vi "new encoder trial.vi"() -> ()   [LabVIEW 2018]
uses:
  <vilib>/Platform/TimedLoop/XDataNode/timing_clust.ctl
  <vilib>/Platform/TimedLoop/XDataNode/nitl_modes.ctl
  <vilib>/Platform/TimedLoop/XDataNode/wakeup.ctl
  <vilib>/rvi/eio/common/nirviEmuTemplateMethod_errors.vi
  <vilib>/rvi/Emulation/niFpgaGetClockAttributes.vi
  <vilib>/rvi/Emulation/niFpgaSctlEmulationGetInTimedLoop.vi
  <vilib>/rvi/Emulation/niFpgaEmulationReportErrorSimple.vi
  <vilib>/rvi/Emulation/niFpgaCriticalErrorInLSC.vi
  <vilib>/eio/EIOMethodNode/EIOMethodNode.xnode
  <vilib>/eio/EIONode/EIONode.xnode
  <vilib>/platform/TimedLoop/XDataNode/XDataNode.xnode
  <vilib>/Platform/TimedLoop/XDataNode/XDNodeRunTimeDep.lvlib
panel:
  out "Mod7/DIO1":bool
  out "Mod7/DIO0":bool
  out "appended array":sgl[](array[numeric])
  out "edge detected":bool
  in  "falling edge (F)":bool caption="Torque encoder direction"
  in  "switch encoders":bool
  in  "filterTorque":bool
  in  "encoders offset":sgl caption="encoder offset (radians)"
  in  "Digital Out":bool[](array[boolean])=[FALSE, FALSE, FALSE, FALSE, FALSE, FALSE, FALSE, FALSE]
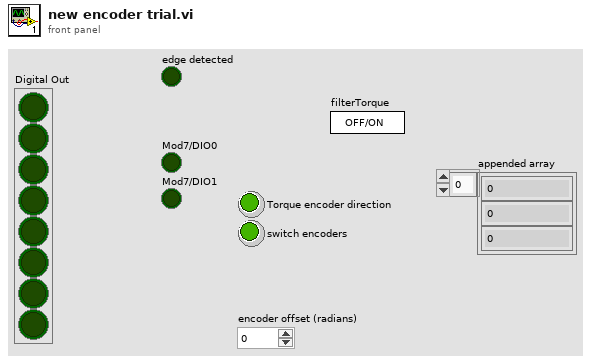
[diagram p1: front panel]
types:
  T1 = typedef "XDNodeRunTimeDep.lvlib/timing_clust.ctl" = cluster{"Expected End [f-1]":u64, "Actual End [f-1]":u64, "Finished Late? [f-1]":bool, "Expected End [i-1]":u64, "Actual End [i-1]":u64, "Finished Late? [i-1]":bool, "Expected Start [i]":u64, "Actual Start [i]":u64, "Expected Start [f]":u64, "Actual Start [f]":u64, "Source Name":string, "Structure Name":string, "Period":i64, "Deadline":i64, "Offset":i64, "Start":i64, "Priority":i32, "Timeout":i32, "Mode":T2, "Wakeup Reason":T3, "Error":errorcluster, "Source Type":string, "Secondary Source Type":string, "Global End Time":u64, "Global Start Time":u64, "Frame Duration":u64, "Iteration Duration":u64, "Assigned CPU":i32, "I/O Scan Engine Mode":u32}
  T2 = typedef "XDNodeRunTimeDep.lvlib/nitl_modes.ctl" = enum32{"No Change", "Process missed periods, maintain original phase", "Discard missed periods, maintain original phase", "Process missed periods, ignore original phase", "Discard missed periods, ignore original phase"}
  T3 = typedef "XDNodeRunTimeDep.lvlib/wakeup.ctl" = enum32{"Normal", "Aborted", "Asynchronous wakeup", "Timing source error", "Timed loop error", "Timeout"}
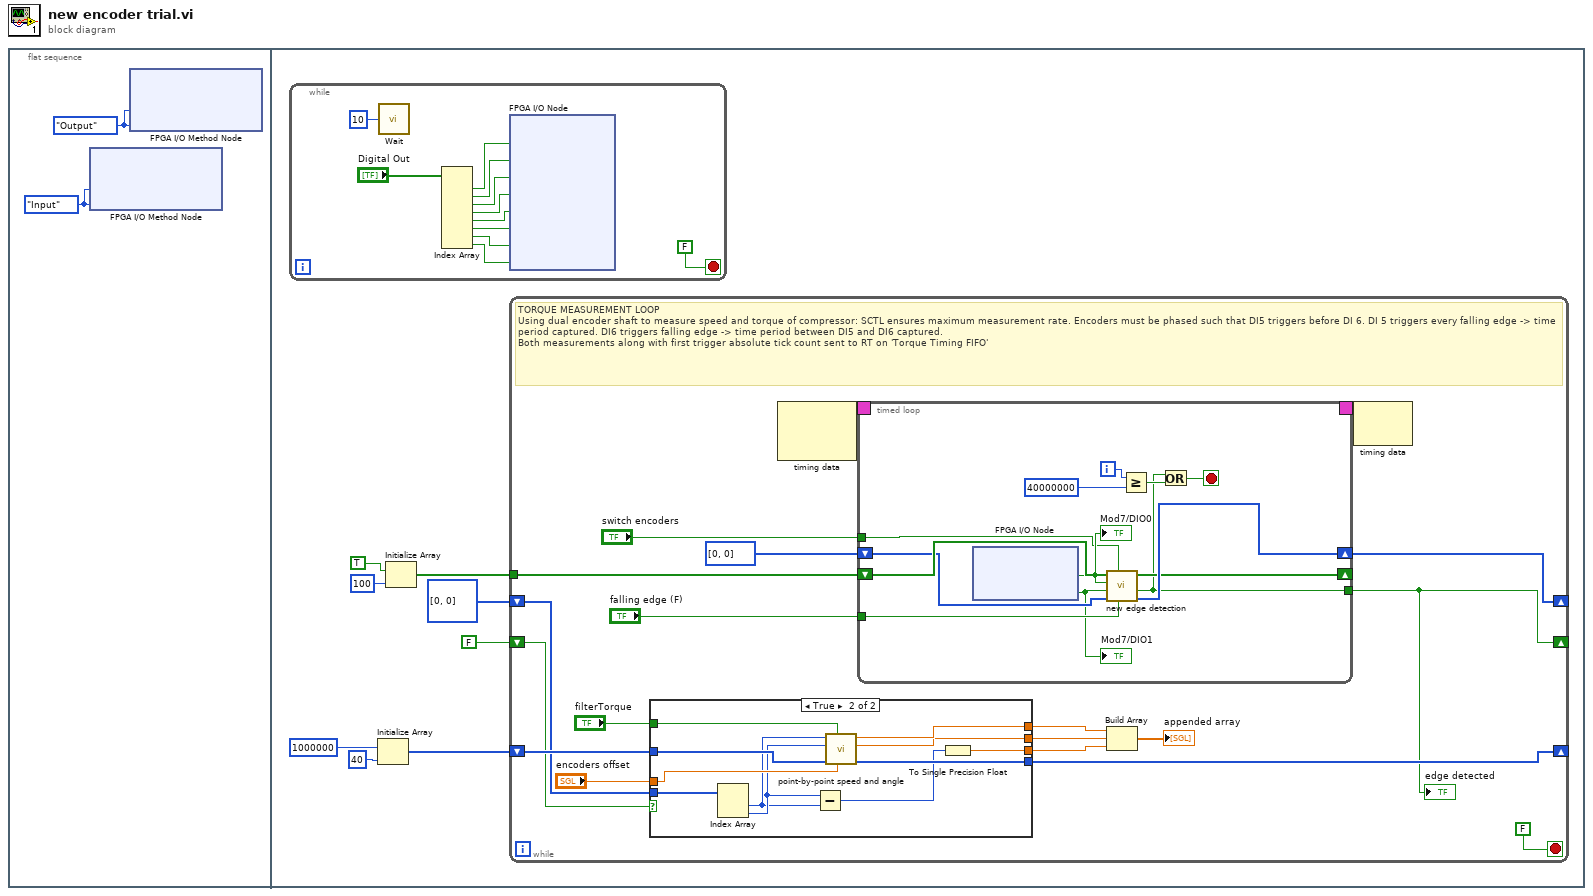
[diagram p0: block diagram]
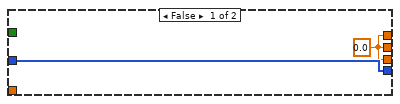
[diagram p2: hidden frame]
diagram:
  n1 = flat-sequence {
    frame #0 {
      w2 = enum8{"No Change", "Input", "Output"}."Input" ("DIO 7:4")
      w1 = enum8{"No Change", "Input", "Output"}."Output" ("DIO 7:4")
      n2 = xnode "FPGA I/O Method Node"("DIO 7:4"=w2, "DIO 3:0"=w2) -> ()  [unwired: 1 in, 1 out]
      n3 = xnode "FPGA I/O Method Node"("DIO 7:4"=w1, "DIO 3:0"=w1) -> ()  [unwired: 1 in, 1 out]
    }
    frame #1 {
      n4 = while {
        stop <- FALSE stop-if-true
        n5 = call "Wait"("Count(mSec)"=u8 10) -> ()  [unwired: 1 out]
        n6 = Index Array(array="Digital Out") -> (element #1=w62:bool, element #2=w63:bool, element #3=w64:bool, element #4=w65:bool, element #5=w66:bool, element #6=w67:bool, element #7=w68:bool, element #8=w69:bool)  [unwired: 8 in]
        n7 = xnode "FPGA I/O Node"("Mod8/DIO0"=w62, "Mod8/DIO1"=w63, "Mod8/DIO2"=w64, "Mod8/DIO3"=w65, "Mod8/DIO4"=w66, "Mod8/DIO5"=w67, "Mod8/DIO6"=w68, "Mod8/DIO7"=w69) -> ()  [unwired: 8 in, 8 out]
      }
      n8 = Initialize Array(u32 1000000 ("64bit integer"), 40 ("dimension size")) -> (w9:u32[])
      n9 = Initialize Array(TRUE, 100 ("edge buffer size")) -> (w10:bool[])
      n10 = while {
        shift-right: [w27] -> _
        shift-left: w9 -> [w28]
        tunnel: w10 -> [w26]
        shift-right: [w15] -> _
        shift-left: u32[] [0, 0] ("step") -> [w14]
        shift-right: [w12] -> _
        shift-left: FALSE ("edge detected") -> [w13]
        stop <- FALSE stop-if-true
        # "TORQUE MEASUREMENT LOOP\nUsing dual encoder shaft to measure speed and torque of compressor: SCTL ensures maximum measurement rate. Encoders must be phased such that DI5 triggers before DI 6. DI 5 triggers every falling edge -> time period captured. DI6 triggers falling edge -> time period between DI5 and DI6 captured.\nBoth measurements along with first trigger absolute tick count sent to RT on 'Torque Timing FIFO'"
        n11 = case shown="True" w13 {
          tunnel: w28 -> [w31 w42]
          tunnel: [w31 w41] -> w27
          tunnel: [w30 w40] -> w20
          tunnel: [w30 w39] -> w17
          tunnel: w14 -> [_ w38]
          tunnel: "encoders offset" -> [_ w37]
          tunnel: "filterTorque" -> [_ w36]
          tunnel: [w30 w32] -> w16
          frame False {
            w30 = sgl 0.0 ("calculated speed (Hz)")
          }
          frame True {
            n12 = Index Array(array=w38) -> (element #1=w34:u32, element #2=w35:u32)  [unwired: 2 in]
            n13 = Subtract(x=w35, y=w34) -> (x-y=w33:u32)
            n14 = call "point-by-point speed and angle.vi"("encoder fixed offest"=w37, "filter torque"=w36, "speed history in"=w42, "angle pulse"=w35, "speed pulse"=w34) -> ("speed history out"=w41:u32[], "calculated angle (radians)"=w39:sgl, "calculated speed (rad/tick)"=w40:sgl)  [unwired: 4 in]
            n15 = To Single Precision Float(number=w33) -> (single precision float=w32:sgl)
          }
        }
        n16 = node-c288() -> (w24:T1)  [unwired: 2 in]
        n17 = timed-loop {
          timing: w24 -> [_]
          timing-out: [_] -> w23
          shift-right: [w49] -> _
          shift-left: w26 -> [w52]
          shift-right: [w50] -> w15
          shift-left: u32[] [0, 0] ("step") -> [w51]
          tunnel: "falling edge (F)" -> [w46]
          tunnel: [w47] -> w12
          tunnel: "switch encoders" -> [w43]
          i -> [w55]
          stop <- w48 stop-if-true
          n18 = xnode "FPGA I/O Node"() -> ("Mod7/DIO0"=w45:bool, "Mod7/DIO1"=w44:bool)  [unwired: 2 in, 2 out]
          "Mod7/DIO0" <- w45
          "Mod7/DIO1" <- w44
          n19 = call "new edge detection.vi"("rising edge (T)"=w46, "switch encoders (F)"=w43, "ticks"=w51, "encoder 2"=w44, "encoder 1"=w45, "history in"=w52) -> ("ticks out"=w50:u32[], "edge detected"=w47:bool, "history out"=w49:bool[])  [unwired: 3 in]
          n20 = Greater Or Equal?(x=w55, y=40000000) -> (x >= y?=w53:bool)
          n21 = Or(x=w47, y=w53) -> (x .or. y?=w48:bool)
        }
        "edge detected" <- w12
        n22 = Build Array(w20, w17, w16) -> (→"appended array":sgl[])
        n23 = node-c288(w23) -> ()  [unwired: 1 out]
      }
    }
  }
